vi "VisionData.vi"() -> ()   [LabVIEW 2011]
panel:
  in  "VisionDataLocal":T1
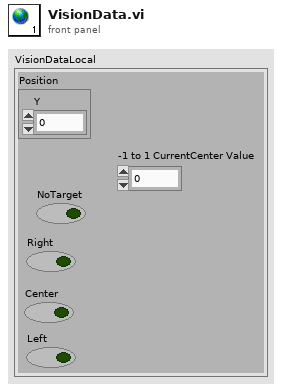
[diagram p1: front panel]
types:
  T1 = cluster{"Position":cluster{"Y":dbl}, "NoTarget":bool, "Right":bool, "Center":bool, "Left":bool, "-1 to 1 CurrentCenter Value":dbl}
diagram:
